vi "Full DMM Scan DER - 2 SCANs.vi"() -> ()   [LabVIEW 2021]
uses:
  DMM SCAN DER/Typedefs/Scan configuration.ctl
  <instrlib>/niDMM/nidmm.llb/niDMM Resolution in Digits.ctl
  DMM SCAN DER/Typedefs/Formatted measurement.ctl
  DMM SCAN DER/Typedefs/Measurement values.ctl
  DMM Mixed Measurements/DMM Mixed Meas Typedefs/DMM Execution Settings.ctl
  DMM SCAN DER/Typedefs/Scan Resource Names.ctl
  <instrlib>/niDMM/nidmm.llb/niDMM Powerline Frequency.ctl
  DMM SCAN DER/DMM_Scan DAQ Ext RLY.lvlib
  DMM Mixed Measurements/DMM_Mixed Measurement.lvlib
panel:
  out "Total Scan Time (s) 2":dbl=0.2938414999998713 format="%#.3p"
  out "Formatted Measurements 2":T1[](array[typedef])=[{"Channel"="ch1", "Switch Time"=0.08098860000018249, "Formatted Measurement"="96.2030mV (dc)", "Out of Range"=FALSE}, {"Channel"="ch2", "Switch Time"=0.1338888999998744, "Formatted Measurement"="9.18027uA (dc)", "Out of Range"=FALSE}, {"Channel"="ch0", "Switch Time"=0.07896019999998316, "Formatted Measurement"="9.89343V (dc)", "Out of Range"=FALSE}] {"Switch Time" format="%#_3p"}
  in  "Scan configuration 2":T2[](array[typedef])=[{"Channel"="ch1", "Resolution in Digits"=5.5, "Range and Function"=enum."DC 100 mV"}, {"Channel"="ch2", "Resolution in Digits"=5.5, "Range and Function"=enum."DC 10 uA"}, {"Channel"="ch0", "Resolution in Digits"=5.5, "Range and Function"=enum."DC 10 V"}] {"Resolution in Digits" items=["3 1/2"=3.5, "4 1/2"=4.5, "5 1/2"=5.5, "6 1/2"=6.5, "7 1/2"=7.5]}
  out "Topology Mapping Output":string[][](array[string])=[["ch0", "Voltage Type", "cDAQ_9477/port0/line0"], ["ch1", "Voltage Type", "cDAQ_9477/port0/line1"], ["ch2", "Current Type ", "cDAQ_9477/port0/line2"], ["ch3", "Shunt Type linked to ch2", "cDAQ_9477/port0/line3"], ["ch4", "", "cDAQ_9477/port0/line4"], ["ch5", "", "cDAQ_9477/port0/line5"], ["ch6", "", "cDAQ_9477/port0/line6"], ["ch7", "", "cDAQ_9477/port0/line7"], ["ch8", "", "cDAQ_9477/port0/line8"], ["ch9", "", "cDAQ_9477/port0/line9"], ["ch10", "", "cDAQ_9477/port0/line10"], ["ch11", "", "cDAQ_9477/port0/line11"], ["ch12", "", "cDAQ_9477/port0/line12"], ["ch13", "", "cDAQ_9477/port0/line13"], ["ch14", "", "cDAQ_9477/port0/line14"], ["ch15", "", "cDAQ_9477/port0/line15"], ["ch16", "", "cDAQ_9477/port0/line16"], ["ch17", "", "cDAQ_9477/port0/line17"], ["ch18", "", "cDAQ_9477/port0/line18"], ["ch19", "", "cDAQ_9477/port0/line19"], ["ch20", "", "cDAQ_9477/port0/line20"], ["ch21", "", "cDAQ_9477/port0/line21"], ["ch22", "", "cDAQ_9477/port0/line22"], ["ch23", "", "cDAQ_9477/port0/line23"], ["ch24", "", "cDAQ_9477/port0/line24"], ["ch25", "", "cDAQ_9477/port0/line25"], ["ch26", "", "cDAQ_9477/port0/line26"], ["ch27", "", "cDAQ_9477/port0/line27"], ["ch28", "", "cDAQ_9477/port0/line28"], ["ch29", "", "cDAQ_9477/port0/line29"], ["ch30", "", "cDAQ_9477/port0/line30"], ["ch31", "", "cDAQ_9477/port0/line31"]]
  in  "error in":errorcluster
  in  "Relays Debounce Time (ms)":u32=5
  in  "Close all Shunts?":bool=TRUE
  in  "Channels Topology Mapping":T4={"Min Channel Voltage"=0, "Max Channel Voltage"=1, "Min Channel Current"=2, "Max Channel Current"=2, "N Shift Shunt to Min Channel Current"=1} caption="Channels Topology mapping"
  in  "Powerline Frequency":T5=enum."50 Hz"
  in  "Scan Resource Names":T6={"DMM Resource Name"="DMM_4065", "DAQ Resource Physical Channels Names"="cDAQ_9477/port0/line0:31"} caption="Scan Resources Names"
  out "Total Scan Time (s)":dbl=0.4171314000000166 format="%#.3p"
  out "Execution Settings":T7[](array[typedef])=[{"Absolute\nResolution"=-1e-05, "Input Resistance\n(Ohm)"=10000000.0, "Digits\nResolution"=5.5, "Range"=-1.0, "Minimum\nFrequency (Hz)"=20.0, "Aperture\nTime (s)"=0.003333333333333333, "Auto Range\nValue"=10.0, "Settle\nTime (s)"=-1.0, "Function"=1}, {"Absolute\nResolution"=-1e-05, "Input Resistance\n(Ohm)"=10000000.0, "Digits\nResolution"=5.5, "Range"=-1.0, "Minimum\nFrequency (Hz)"=20.0, "Aperture\nTime (s)"=0.003333333333333333, "Auto Range\nValue"=0.1, "Settle\nTime (s)"=-1.0, "Function"=1}, {"Absolute\nResolution"=-1e-05, "Input Resistance\n(Ohm)"=-1.0, "Digits\nResolution"=5.5, "Range"=-1.0, "Minimum\nFrequency (Hz)"=20.0, "Aperture\nTime (s)"=0.003333333333333333, "Auto Range\nValue"=0.01, "Settle\nTime (s)"=-1.0, "Function"=3}] {"Function" items=["DC Volts"=1, "AC Volts"=2, "DC Current"=3, "AC Current"=4, "2-Wire Resistance"=5, "4-Wire Resistance"=101, "Frequency"=104, "Period"=105, "AC Volts DC Coupled"=1001, "Diode"=1002, "Waveform Voltage"=1003, "Waveform Current"=1004, "Capacitance"=1005, "Inductance"=1006, "Temperature"=108]; "Absolute\nResolution" format="%#_6p"; "Input Resistance\n(Ohm)" format="%#_6p"; "Range" format="%#_6p"; "Minimum\nFrequency (Hz)" format="%#_6p"; "Aperture\nTime (s)" format="%#_6p"; "Auto Range\nValue" format="%#_6p"; "Settle\nTime (s)" format="%#_6p"}
  out "Raw Measurements":T8[](array[typedef])=[{"Channel"="ch0", "Value"=9.895307782234099, "Unit"="V (dc)", "Out of Range"=FALSE}, {"Channel"="ch1", "Value"=0.09756682204953278, "Unit"="V (dc)", "Out of Range"=FALSE}, {"Channel"="ch2", "Value"=9.225803040924296e-06, "Unit"="A (dc)", "Out of Range"=FALSE}] {"Value" format="%#_8g"}
  out "Formatted Measurements":T1[](array[typedef])=[{"Channel"="ch0", "Switch Time"=0.11334120000037728, "Formatted Measurement"="9.89531V (dc)", "Out of Range"=FALSE}, {"Channel"="ch1", "Switch Time"=0.11394489999975121, "Formatted Measurement"="97.5668mV (dc)", "Out of Range"=FALSE}, {"Channel"="ch2", "Switch Time"=0.18984110000019427, "Formatted Measurement"="9.22580uA (dc)", "Out of Range"=FALSE}] {"Switch Time" format="%#_3p"}
  in  "Scan configuration":T2[](array[typedef])=[{"Channel"="ch0", "Resolution in Digits"=5.5, "Range and Function"=enum."DC Voltage Auto Range"}, {"Channel"="ch1", "Resolution in Digits"=5.5, "Range and Function"=enum."DC Voltage Auto Range"}, {"Channel"="ch2", "Resolution in Digits"=5.5, "Range and Function"=enum."DC Current Auto Range"}] {"Resolution in Digits" items=["3 1/2"=3.5, "4 1/2"=4.5, "5 1/2"=5.5, "6 1/2"=6.5, "7 1/2"=7.5]}
  out "error out":errorcluster
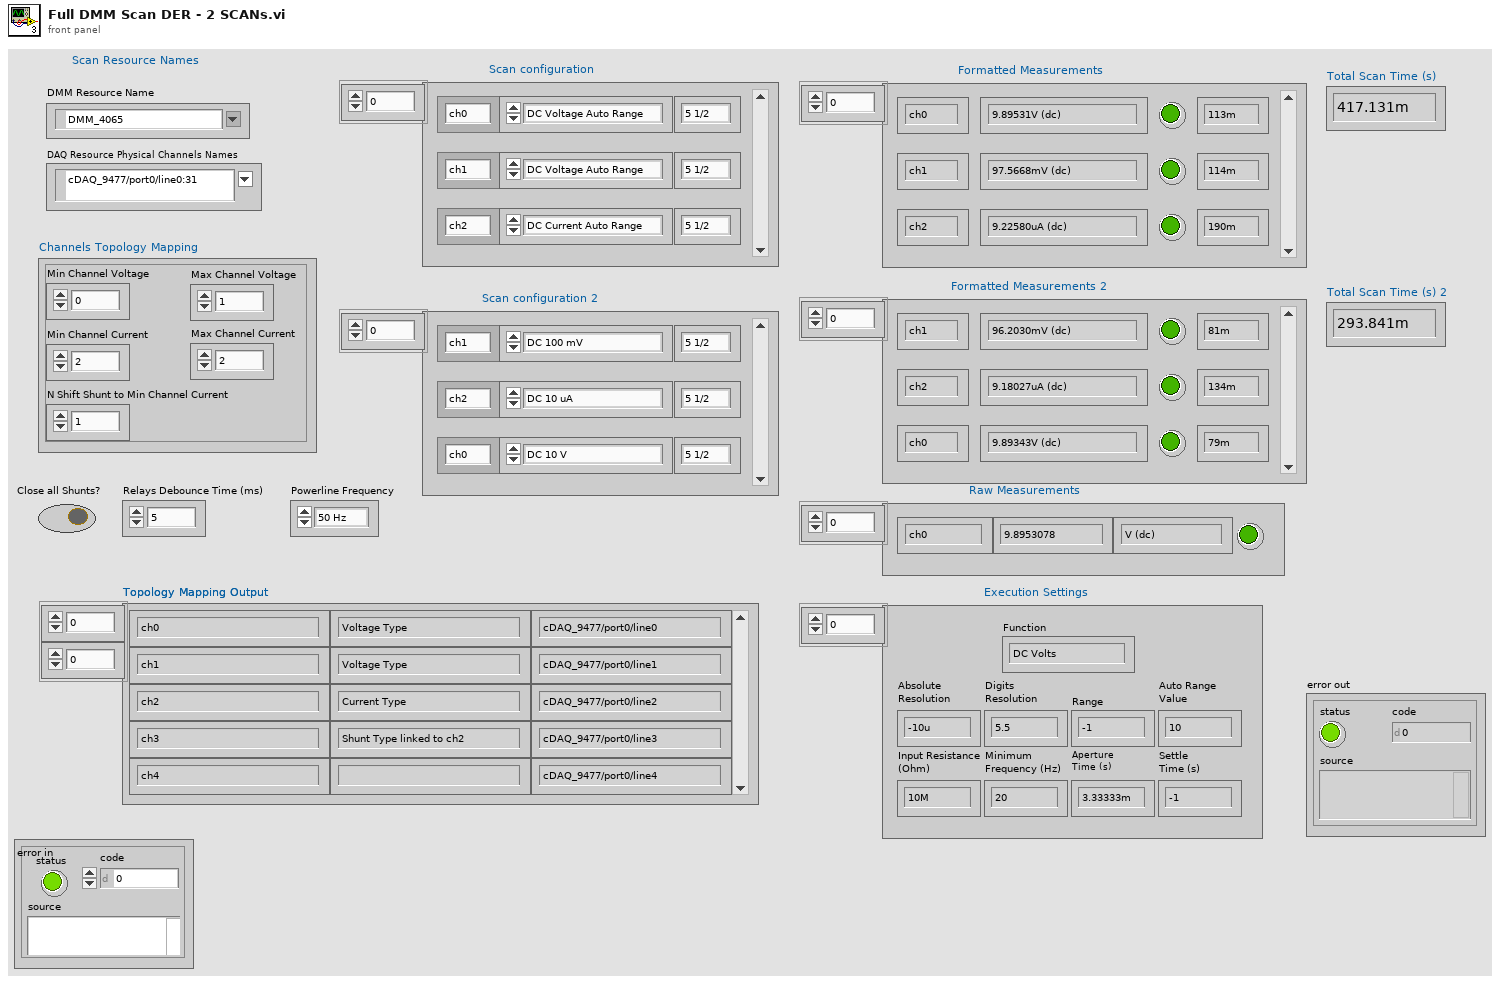
[diagram p1: front panel]
types:
  T1 = typedef "DMM_Scan DAQ Ext RLY.lvlib/Formatted measurement.ctl" = cluster{"Channel":string, "Switch Time":dbl, "Formatted Measurement":string, "Out of Range":bool}
  T2 = typedef "DMM_Scan DAQ Ext RLY.lvlib/Scan configuration.ctl" = cluster{"Channel":string, "Resolution in Digits":T3, "Range and Function":enum16{"DC Voltage Auto Range", "DC 100 mV", "DC 1 V ", "DC 10 V", "DC 100 V", "DC 300 V", " ", "AC Voltage Auto Range", "AC 50 mV", "AC 200 mV", "AC 500 mV", "AC 2 V", "AC 5 V", "AC 20 V", "AC 50 V", "AC 300 V", "  ", "DC Current Auto Range", "DC 1 uA", "DC 10 uA", "DC 100 uA", "DC 1 mA", "DC 10 mA", "DC 20 mA", "DC 100 mA", "DC 200 mA", "DC 1 A", "DC 3 A", "   ", "AC Current Auto Range", "AC 100 uA", "AC 1 mA", "AC 10 mA", "AC 100 mA", "AC 500 mA", "AC 1 A", "AC 3 A", "    ", "Resistance Auto Range", "Res 100 Ohm", "Res 1 kOhm", "Res 10 kOhm", "Res 100 kOhm", "Res 1 MOhm", "Res 10 MOhm", "Res 100 MOhm", "Res 5 GOhm", "     ", "Frequency AC Auto Range", "Freq AC 50 mV", "Freq AC 500 mV", "Freq AC 5 V", "Freq AC 50 V", "Freq AC 300 V", "      ", "Period AC Auto Range", "Period AC 50 mV", "Period AC 500 mV", "Period AC 5 V", "Period AC 50 V", "Period AC 300 V"}}
  T3 = typedef "niDMM Resolution in Digits.ctl" = dbl
  T4 = cluster{"Min Channel Voltage":u32, "Max Channel Voltage":u32, "Min Channel Current":u32, "Max Channel Current":u32, "N Shift Shunt to Min Channel Current":u32}
  T5 = typedef "niDMM Powerline Frequency.ctl" = enum16{"60 Hz", "50 Hz"}
  T6 = typedef "DMM_Scan DAQ Ext RLY.lvlib/Scan Resource Names.ctl" = cluster{"DMM Resource Name":refnum<k15>, "DAQ Resource Physical Channels Names":tag}
  T7 = typedef "DMM_Mixed Measurement.lvlib/DMM Execution Settings.ctl" = cluster{"Absolute\nResolution":dbl, "Input Resistance\n(Ohm)":dbl, "Digits\nResolution":dbl, "Range":dbl, "Minimum\nFrequency (Hz)":dbl, "Aperture\nTime (s)":dbl, "Auto Range\nValue":dbl, "Settle\nTime (s)":dbl, "Function":i32}
  T8 = typedef "DMM_Scan DAQ Ext RLY.lvlib/Measurement values.ctl" = cluster{"Channel":string, "Value":dbl, "Unit":string, "Out of Range":bool}
  T9 = typedef "DMM_Scan DAQ Ext RLY.lvlib/Scan Resource Handles Out.ctl" = cluster{"DMM Handle":refnum<k15>, "DAQmx Task Out":refnum<k21>, "Relays Status Array":bool[], "N Shift Shunt":u32, "Close all Shunts?":bool, "Relays Debounce Time (ms)":u32}
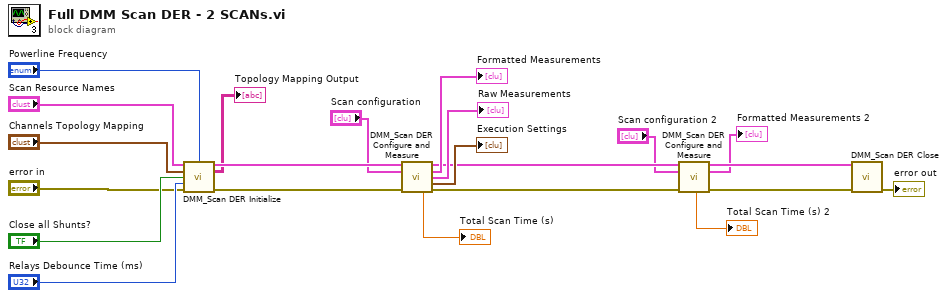
[diagram p0: block diagram]
diagram:
  n1 = call "DMM_Scan DER Initialize.vi"("Scan Resources Names"="Scan Resource Names", "Powerline Frequency"="Powerline Frequency", "Channels Topology Mapping"="Channels Topology Mapping", "Close all Shunts?"="Close all Shunts?", "Relays Debounce Time (ms)"="Relays Debounce Time (ms)", "error in"="error in") -> ("Scan Resources Handles Out"=w21:T9, "Topology Mapping Output"=→"Topology Mapping Output":string[][], "error out"=w22:errorcluster)  [unwired: 7 in]
  n2 = call "DMM_Scan DER Configure and Measure.vi"("Scan Resources Handles In"=w21, "Scan Configuration"="Scan configuration", "error in"=w22) -> ("Scan Resources Handles Out"=w5:T9, "Formatted Measurements"=→"Formatted Measurements":T1[], "Raw Measurements"=→"Raw Measurements":T8[], "Execution Settings"=→"Execution Settings":T7[], "Total Scan Time (s)"=→"Total Scan Time (s)":dbl, "error out"=w7:errorcluster)  [unwired: 7 in]
  n3 = call "DMM_Scan DER Configure and Measure.vi"("Scan Resources Handles In"=w5, "Scan Configuration"="Scan configuration 2", "error in"=w7) -> ("Scan Resources Handles Out"=w4:T9, "Formatted Measurements"=→"Formatted Measurements 2":T1[], "Total Scan Time (s)"=→"Total Scan Time (s) 2":dbl, "error out"=w6:errorcluster)  [unwired: 7 in, 2 out]
  n4 = call "DMM_Scan DER Close.vi"("Scan Resources Handles In"=w4, "error in"=w6) -> ("error out"=→"error out":errorcluster)  [unwired: 13 in]
